vi "autonomous mode.vi"() -> ()   [LabVIEW 2012, in "Omni2013.lvrbt"]
uses:
  Omni2013.lvrbt
  <vilib>/NXT/Hardware/Plugins/Tetrix 180 deg Servo/Tetrix180ServoAddress.ctl
  <vilib>/NXT/Hardware/Plugins/Tetrix DC Motor/TetrixDCMotorAddress.ctl
  <vilib>/NXT/HiTechnic/HiTechnic Controls/HiTechnic Port.ctl
  <vilib>/NXT/Block Support/NXT_InputPort.ctl
  <vilib>/NXT/Dual Mode Library/Waits/Wait_Num(msec).vi
  <vilib>/NXT/NXTIO Xnodes/NXTIONodeSubVIs/TETRIX IO Move Servos.vi
  <vilib>/NXT/NXTIO Xnodes/NXTIONodeSubVIs/TETRIX IO Move DC Motors.vi
  <vilib>/NXT/HiTechnic/HiTechnic Config/HiTechnic IRSeeker Mode1200Hz.vi
  <vilib>/NXT/HiTechnic/HiTechnic SubVIs/HiTechnic IRSeeker Sensor_AC dir.vi
  <vilib>/NXT/Dual Mode Library/Sensors/Sonar_cm.vi
  <vilib>/NXT/Dual Mode Library/Display/drawNumber.vi
  <vilib>/NXT/HiTechnic/HiTechnic Read/HiTechnic IRSeeker Sensor_AC all.vi
  <vilib>/NXT/NXTIO Xnodes/AddressXNode/NXTIOAddress.xnode
  <vilib>/NXT/NXTIO Xnodes/NXTIOXNode/NXTIO.xnode
  <vilib>/NXT/Subs/LVHSConnector.ctl
  <vilib>/NXT/LegoClasses/BrickReference/BrickReference.lvclass
panel:
  in  "Translation U&D":dbl
  in  "Translation L&R":dbl
  in  "Rotation":dbl
  out "Enabled":bool
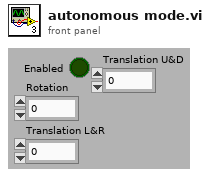
[diagram p1: front panel]
types:
  T1 = typedef "LVHSConnector.ctl" = refnum<class "BrickReference.lvclass">
  T2 = typedef "HiTechnic Port.ctl" = cluster{"Port":T3, "MUX Port":u8}
  T3 = typedef "NXT_InputPort.ctl" = u8
  T4 = typedef "TetrixDCMotorAddress.ctl" = i16
  T5 = cluster{"TetrixDCMotor":T4, "TetrixDCMotor 2":T4}
  T6 = cluster{"Direction (0-9)":i16, "Signal Strength (Array)":u8[]}
  T7 = typedef "Tetrix180ServoAddress.ctl" = i16
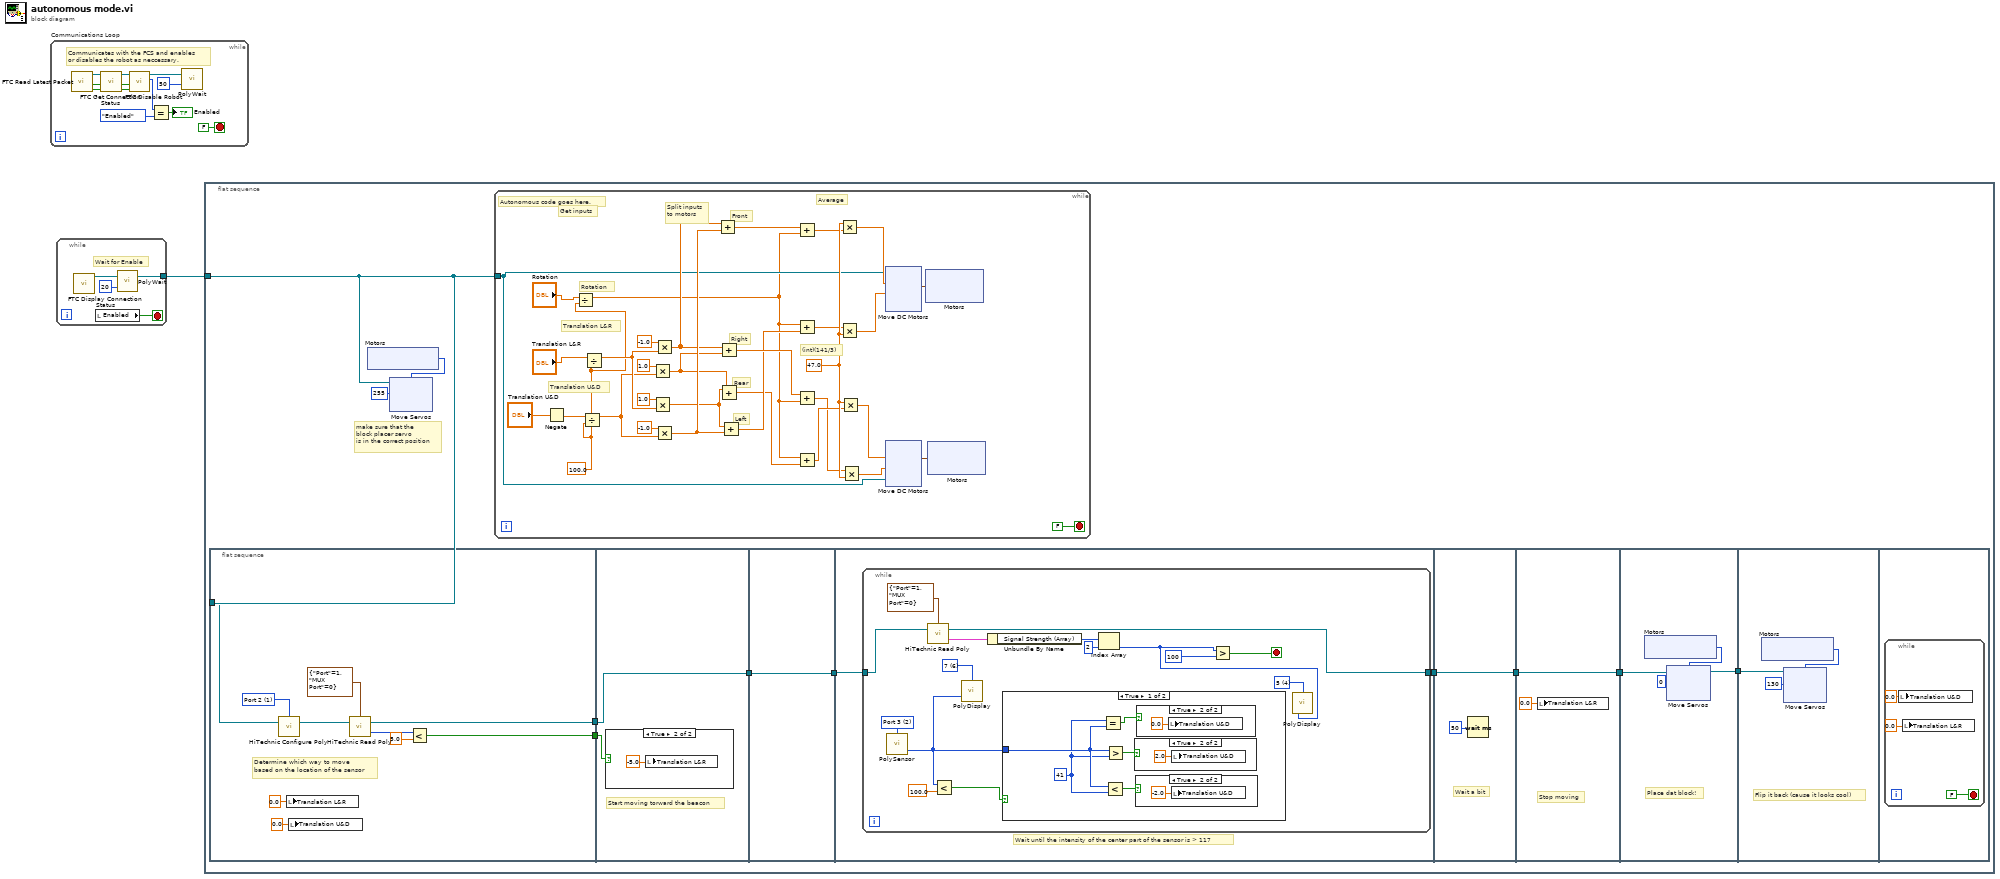
[diagram p0: block diagram]
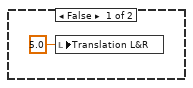
[diagram p2: hidden frame]
diagram:
  n1 = while "Communications Loop" {
    stop <- FALSE stop-if-true
    # "Communicates with the FCS and enables \nor disables the robot as neccessary."
    n2 = call <vilib>:"FTC Read Latest Packet.vi"() -> ("Packet Received?"=w11:bool, "Stopped?"=w10:bool, "NXT"=w13:T1)  [unwired: 6 in, 3 out]
    n3 = call <vilib>:"FTC Get Connection Status.vi"("Packet Received?"=w11, "Stopped?"=w10, "NXT"=w13) -> ("Online?"=w2:bool, "Stopped?"=w3:bool, "NXT"=w12:T1)  [unwired: 5 in]
    n4 = call <vilib>:"FTC Disable Robot.vi"("Online?"=w2, "Stopped?"=w3, "NXT"=w12) -> ("Enabled?"=w6:enum16{"Disabled", "Enabled"}, "NXT"=w8:T1)  [unwired: 3 in]
    n5 = Equal?(x=w6, y=enum16{"Disabled", "Enabled"}."Enabled") -> (x = y?=→"Enabled":bool)
    n6 = call-poly <vilib>:"PolyWait.vi"("Time (100 msec)"=u32 50 ("Time (msec)"), "NXT"=w8) -> ()  [unwired: 2 in, 1 out]
  }
  n7 = while {
    tunnel: [w15] -> w1
    stop <- w16 stop-if-true
    # "Wait for Enable"
    n8 = call <vilib>:"FTC Display Connection Status.vi"() -> ("NXT"=w14:T1)  [unwired: 11 in]
    n9 = local read "Enabled"() -> (w16:bool)
    n10 = call-poly <vilib>:"PolyWait.vi"("Time (100 msec)"=u32 20 ("Time (msec)"), "NXT"=w14) -> ("NXT"=w15:T1)  [unwired: 2 in]
  }
  n11 = flat-sequence {
    tunnel: w1 -> [w26]
    frame #0 {
      # "make sure that the \nblock placer servo \nis in the correct position"
      n12 = flat-sequence {
        tunnel: [w41] -> w21
        tunnel: w26 -> [w37]
        tunnel: [w40] -> w20
        tunnel: w21 -> [w47]
        tunnel: [w48] -> w19
        tunnel: w20 -> [w48]
        tunnel: w19 -> [w51]
        tunnel: [w51] -> w18
        tunnel: w18 -> [w53]
        tunnel: [w52] -> w23
        tunnel: w23 -> [w78]
        tunnel: [w78] -> w22
        tunnel: [w79] -> w25
        tunnel: w22 -> [w79]
        tunnel: w25 -> [w82]
        tunnel: [w81] -> w24
        tunnel: w24 -> [w93]
        frame #0 {
          w42 = T3 1 items=["Port 1", "Port 2", "Port 3", "Port 4"] ("Port")
          # "Determine which way to move \nbased on the location of the sensor"
          n13 = call-poly <vilib>:"HiTechnic Configure Poly.vi"("NXT"=w37, "Port"=w42) -> ("NXT"=w43:T1)  [unwired: 2 in]
          n14 = local write "Translation L&R"(0.0 ("Translation L&R")) -> ()
          n15 = local write "Translation U&D"(0.0 ("Translation U&D")) -> ()
          n16 = call-poly <vilib>:"HiTechnic Read Poly.vi"("NXT"=w43, "Port/MUX"=T2 {"Port"=1, "MUX Port"=0}) -> ("Direction (0-9)"=w44:i16, "NXT"=w40:T1)  [unwired: 1 in]
          n17 = Less?(x=w44, y=5.0) -> (x < y?=w41:bool)
        }
        frame #1 {
          # "Start moving torward the beacon"
          n18 = case shown="True" w47 {
            frame False {
              n19 = local write "Translation L&R"(5.0 ("Translation L&R")) -> ()
            }
            frame True {
              n20 = local write "Translation L&R"(-5.0 ("Translation L&R")) -> ()
            }
          }
        }
        frame #2 {
        }
        frame #3 {
          # "Wait until the intensity of the center part of the sensor is > 117"
          n21 = while {
            tunnel: w53 -> [w60]
            tunnel: [w58] -> w52
            stop <- w64 stop-if-true
            w57 = i16 6 items=["1", "2", "3", "4", "5", "6", "7", "8"] ("Line")
            w59 = T3 2 items=["Port 1", "Port 2", "Port 3", "Port 4"] ("Port (Port 4)")
            w63 = i16 4 items=["1", "2", "3", "4", "5", "6", "7", "8"] ("Line")
            n22 = call-poly <vilib>:"PolySensor.vi"("Port (Port 4)"=w59) -> ("Distance (cm)"=w55:i16)  [unwired: 2 in, 1 out]
            n23 = call-poly <vilib>:"HiTechnic Read Poly.vi"("NXT"=w60, "Port/MUX"=T2 {"Port"=1, "MUX Port"=0}) -> ("All Info"=w67:T6, "NXT"=w58:T1)  [unwired: 1 in]
            n24 = Less?(x=w55, y=100.0) -> (x < y?=w54:bool)
            n25 = call-poly <vilib>:"PolyDisplay.vi"("number"=w55, "Line"=w57) -> ()  [unwired: 2 in, 1 out]
            n26 = Unbundle By Name(w67) -> ("Signal Strength (Array)"=w66:u8[])
            n27 = case shown="True" w54 {
              tunnel: w55 -> [w71 _]
              frame True {
                w70 = i16 41 ("y")
                n28 = Equal?(x=w70, y=w71) -> (x = y?=w69:bool)
                n29 = Less?(x=w71, y=w70) -> (x < y?=w73:bool)
                n30 = Greater?(x=w71, y=w70) -> (0:w72:bool)
                n31 = case shown="True" w72 {
                  frame False {
                  }
                  frame True {
                    n32 = local write "Translation U&D"(2.0 ("Translation U&D")) -> ()
                  }
                }
                n33 = case shown="True" w73 {
                  frame False {
                  }
                  frame True {
                    n34 = local write "Translation U&D"(-2.0 ("Translation U&D")) -> ()
                  }
                }
                n35 = case shown="True" w69 {
                  frame False {
                  }
                  frame True {
                    n36 = local write "Translation U&D"(0.0 ("Translation U&D")) -> ()
                  }
                }
              }
              frame False {
              }
            }
            n37 = Index Array(array=w66, index=2) -> (element=w62:u8)
            n38 = Greater?(x=w62, y=u8 100) -> (0:w64:bool)
            n39 = call-poly <vilib>:"PolyDisplay.vi"("number"=w62, "Line"=w63) -> ()  [unwired: 2 in, 1 out]
          }
        }
        frame #4 {
          # "Wait a bit"
          n40 = Wait (ms)(milliseconds to wait=u32 50) -> ()  [unwired: 1 out]
        }
        frame #5 {
          # "Stop moving"
          n41 = local write "Translation L&R"(0.0 ("Translation L&R")) -> ()
        }
        frame #6 {
          # "Place dat block!"
          n42 = xnode "Motors"() -> ("Motor"=w84:T7)
          n43 = xnode "Move Servos"("Position 1"=u8 0, "Servos"=w84, "NXT"=w82) -> ("NXT"=w81:T1)
        }
        frame #7 {
          # "Flip it back (cause it looks cool)"
          n44 = xnode "Motors"() -> ("Motor"=w95:T7)
          n45 = xnode "Move Servos"("Position 1"=u8 130, "Servos"=w95, "NXT"=w93) -> ()  [unwired: 1 out]
        }
        frame #8 {
          n46 = while {
            stop <- FALSE stop-if-true
            n47 = local write "Translation U&D"(0.0 ("Translation U&D")) -> ()
            n48 = local write "Translation L&R"(0.0 ("Translation L&R")) -> ()
          }
        }
      }
      n49 = xnode "Motors"() -> ("Motor"=w28:T7)
      n50 = xnode "Move Servos"("Position 1"=u8 255, "Servos"=w28, "NXT"=w26) -> ()  [unwired: 1 out]
      n51 = while {
        tunnel: w26 -> [w112]
        stop <- FALSE stop-if-true
        w108 = 100.0 ("y")
        w139 = 47.0 ("y")
        # "Average"
        # "Left"
        # "Rear"
        # "Right"
        # "Front"
        # "(int)(141/3)"
        # "Split inputs to motors"
        # "Get inputs"
        # "Translation U&D"
        # "Rotation"
        # "Translation L&R"
        # "Autonomous code goes here."
        n52 = Negate(x="Translation U&D") -> (-x=w107:dbl)
        n53 = Divide(x="Rotation", y=w108) -> (x/y=w109:dbl)
        n54 = Divide(x=w107, y=w108) -> (x/y=w110:dbl)
        n55 = Divide(x="Translation L&R", y=w108) -> (x/y=w111:dbl)
        n56 = Multiply(x=1.0, y=w110) -> (x*y=w133:dbl)
        n57 = Multiply(x=1.0, y=w111) -> (x*y=w122:dbl)
        n58 = Multiply(x=-1.0, y=w111) -> (x*y=w121:dbl)
        n59 = Multiply(x=-1.0, y=w110) -> (x*y=w134:dbl)
        n60 = Add(x=w121, y=w134) -> (x+y=w118:dbl)
        n61 = Add(x=w121, y=w133) -> (x+y=w120:dbl)
        n62 = Add(x=w122, y=w133) -> (x+y=w117:dbl)
        n63 = Add(x=w122, y=w134) -> (x+y=w119:dbl)
        n64 = Add(x=w118, y=w109) -> (x+y=w137:dbl)
        n65 = Add(x=w109, y=w119) -> (x+y=w136:dbl)
        n66 = Add(x=w120, y=w109) -> (x+y=w135:dbl)
        n67 = Add(x=w109, y=w117) -> (x+y=w138:dbl)
        n68 = Multiply(x=w139, y=w137) -> (x*y=w128:dbl)
        n69 = Multiply(x=w136, y=w139) -> (x*y=w129:dbl)
        n70 = Multiply(x=w139, y=w138) -> (x*y=w132:dbl)
        n71 = Multiply(x=w135, y=w139) -> (x*y=w131:dbl)
        n72 = xnode "Motors"() -> ("Motor"=w127:cluster{"TetrixDCMotor":T4, "TetrixDCMotor":T4})
        n73 = xnode "Move DC Motors"("Power/Speed 2"=w129, "Power/Speed 1"=w128, "Motors"=w127, "NXT"=w112) -> ()  [unwired: 1 out]
        n74 = xnode "Motors"() -> ("Motor"=w130:cluster{"TetrixDCMotor":T4, "TetrixDCMotor":T4})
        n75 = xnode "Move DC Motors"("Power/Speed 2"=w131, "Power/Speed 1"=w132, "Motors"=w130, "NXT"=w112) -> ()  [unwired: 1 out]
      }
    }
  }
